vi "cw_exp5.vi"() -> ()   [LabVIEW 2022 SP3]
panel:
  out "波形图":cluster{i32, sgl, dbl[]}(graph)
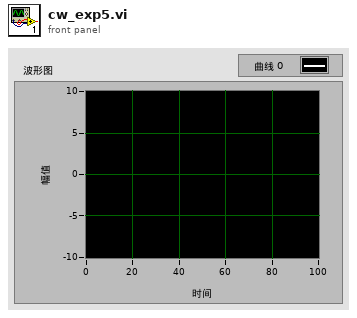
[diagram p1: front panel]
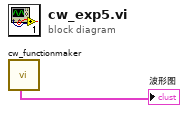
[diagram p0: block diagram]
diagram:
  n1 = call "cw_functionmaker.vi"() -> ("监视器"=→"波形图":cluster{i32, sgl, dbl[]})  [unwired: 10 in, 1 out]
